vi "getCamera.vi"(8 "error in (no error)":errorcluster, 11 "NetworkCamera in":refnum<class "NetworkCamera.lvclass">) -> (0 "error out":errorcluster, 2 "Camera":refnum<class "Camera.lvclass">, 3 "NetworkCamera out":refnum<class "NetworkCamera.lvclass">)   [LabVIEW 2011, in "Hardware.lvlib" / "HWControllers.lvlib" / "NetworkCamera.lvclass"]
uses:
  NetworkCamera.lvclass
  Channels/Camera/Camera/Camera.lvclass
  NetworkCamera.lvclass/NetworkCamera.ctl
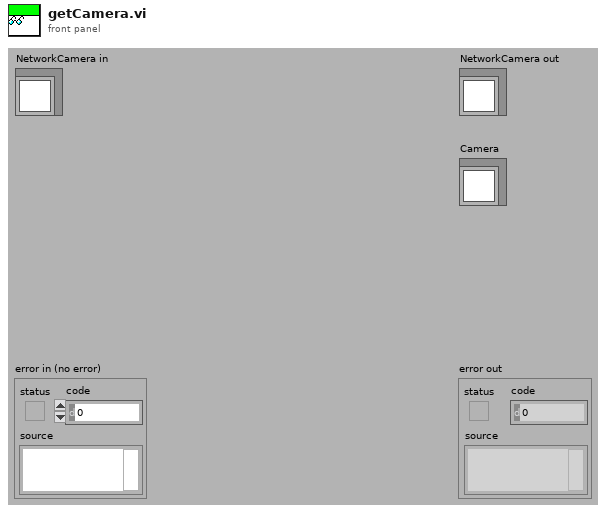
[diagram p1: front panel]
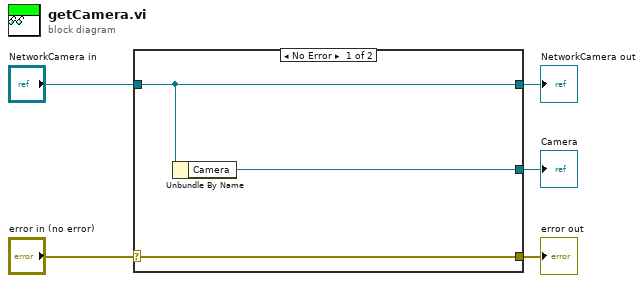
[diagram p0: block diagram]
diagram:
  n1 = case shown="No Error" "error in (no error)" {
    selector: "error in (no error)" -> [w8 w9]
    tunnel: [w8 w9] -> w4
    tunnel: [w7 w10] -> w2
    tunnel: "NetworkCamera in" -> [w7 w10]
    tunnel: [w6 _] -> w1
    frame No Error {
      n2 = Unbundle By Name(w7) -> ("Camera"=w6:refnum<class "Camera.lvclass">)
    }
    frame Error {
    }
  }
  "error out" <- w4
  "NetworkCamera out" <- w2
  "Camera" <- w1
